vi "initialise.vi"(8 "error in (no error)":errorcluster, 11 "MH100301DMC in":refnum<class "StageMH100301DMC.lvclass">) -> (0 "error out":errorcluster, 3 "MH100301DMC out":refnum<class "StageMH100301DMC.lvclass">)   [LabVIEW 2010, in "StageMH100301DMC.lvclass"]
doc: "The dynamic dispatch-version of this VI initalises the plug-in object by allocating and initalising any dynamic resources need."
uses:
  StageMH100301DMC.lvclass
  StageDL090409Scaffold/StageDL090409Scaffold/StageDL090409Scaffold.lvclass
  common/classes/ErrorController/ErrorController/ErrorController.lvclass
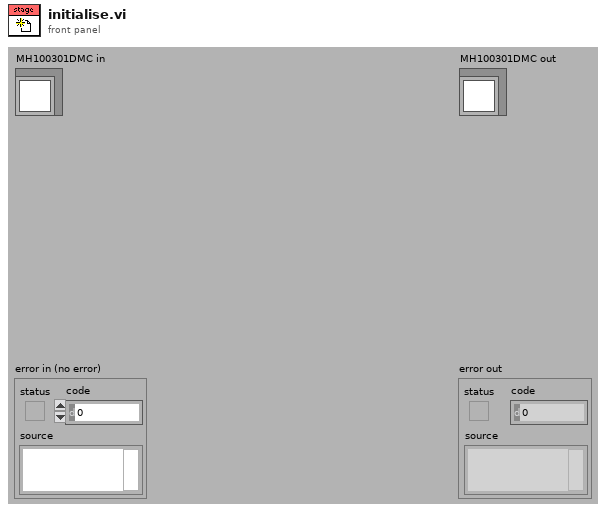
[diagram p1: front panel]
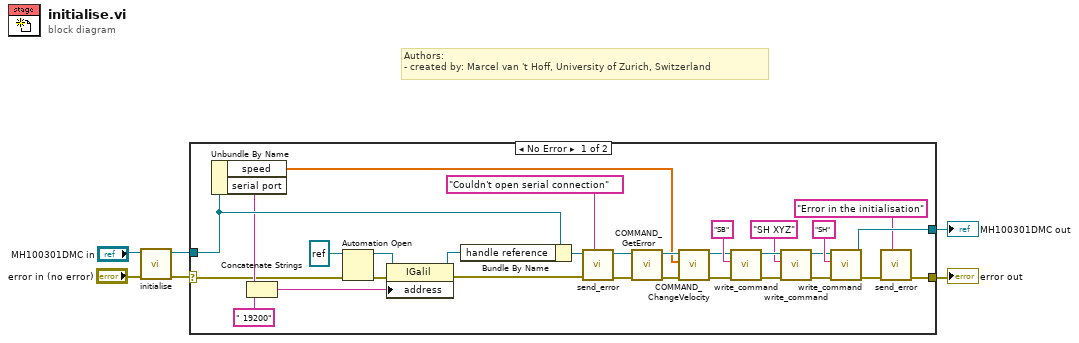
[diagram p0: block diagram]
diagram:
  # "Authors: \n- created by: Marcel van 't Hoff, University of Zurich, Switzerland"
  n1 = call-parent "initialise.vi"("error in (no error)"="error in (no error)", "GenericPlugin in"="MH100301DMC in") -> ("error out"=w4:errorcluster, "GenericPlugin out"=w3:refnum<class "StageMH100301DMC.lvclass">)  [unwired: 8 out]
  n2 = case shown="No Error" w4 {
    selector: w4 -> [w12 w37]
    tunnel: w3 -> [w35 w36]
    tunnel: [w22 w37] -> w2
    tunnel: [w25 w36] -> w1
    frame No Error {
      n3 = Unbundle By Name(w35) -> ("speed"=w31:dbl[unit][], "serial port"=w15:string)
      n4 = Concatenate Strings(w15, " 19200" ("string")) -> (w11:string)
      n5 = Automation Open(error in (no error)=w12, Automation Refnum=refnum<k7> refnum ("Galil.IGalil")) -> (Automation Refnum=w10:refnum<k7>, error out=w9:errorcluster)  [unwired: 2 in]
      n6 = property class="IGalil"(reference=w10, error in=w9, "address"=w11) -> (reference out=w7:refnum<k7>, error out=w8:errorcluster)
      n7 = Bundle By Name(cluster=w35, "handle reference"=w7) -> (w34:refnum<class "StageMH100301DMC.lvclass">)
      n8 = call "send_error.vi"("additional message"="Couldn't open serial connection", "error in (no error)"=w8) -> ("error out"=w21:errorcluster)  [unwired: 9 in]
      n9 = call-dynamic "COMMAND_GetError.vi"("error in (no error)"=w21, "StageMH100301DMC in"=w34) -> ("error out"=w33:errorcluster, "StageMH100301DMC out"=w32:refnum<class "StageMH100301DMC.lvclass">)  [unwired: 8 in]
      n10 = call-dynamic "COMMAND_ChangeVelocity.vi"("error in (no error)"=w33, "configuration data.speed"=w31, "MH100301DMC in"=w32) -> ("error out"=w17:errorcluster, "MH100301DMC out"=w18:refnum<class "StageMH100301DMC.lvclass">)  [unwired: 7 in]
      n11 = call-dynamic "write_command.vi"("error in (no error)"=w17, "command (without terminating \"\\n\")"="SB" ("command (without terminating \"\\n\")"), "MH100301DMC in"=w18) -> ("error out"=w30:errorcluster, "MH100301DMC out"=w29:refnum<class "StageMH100301DMC.lvclass">)  [unwired: 5 in, 2 out]
      n12 = call-dynamic "write_command.vi"("error in (no error)"=w30, "command (without terminating \"\\n\")"="SH XYZ" ("command (without terminating \"\\n\")"), "MH100301DMC in"=w29) -> ("error out"=w24:errorcluster, "MH100301DMC out"=w23:refnum<class "StageMH100301DMC.lvclass">)  [unwired: 5 in, 2 out]
      n13 = call-dynamic "write_command.vi"("error in (no error)"=w24, "command (without terminating \"\\n\")"="SH" ("command (without terminating \"\\n\")"), "MH100301DMC in"=w23) -> ("error out"=w16:errorcluster, "MH100301DMC out"=w25:refnum<class "StageMH100301DMC.lvclass">)  [unwired: 5 in, 2 out]
      n14 = call "send_error.vi"("additional message"="Error in the initialisation", "error in (no error)"=w16) -> ("error out"=w22:errorcluster)  [unwired: 9 in]
    }
    frame Error {
    }
  }
  "error out" <- w2
  "MH100301DMC out" <- w1
